vi "STOP.vi"(8 "error in (no error)":errorcluster, 11 "Stop in":refnum<class "Emulate.lvclass">) -> (0 "error out":errorcluster, 3 "Stop out":refnum<class "Emulate.lvclass">)   [LabVIEW 2019, in "Emulate.lvclass"]
uses:
  Emulate.lvclass
  C:/Users/elysium/Documents/dev/TRANCON/Classes/GeneralFunctionality/GeneralFunctionality.lvclass
  GeneralFunctionality/GeneralFunctionality.lvclass/GeneralFunctionality.ctl
  GeneralFunctionality/GeneralFunctionality.lvclass
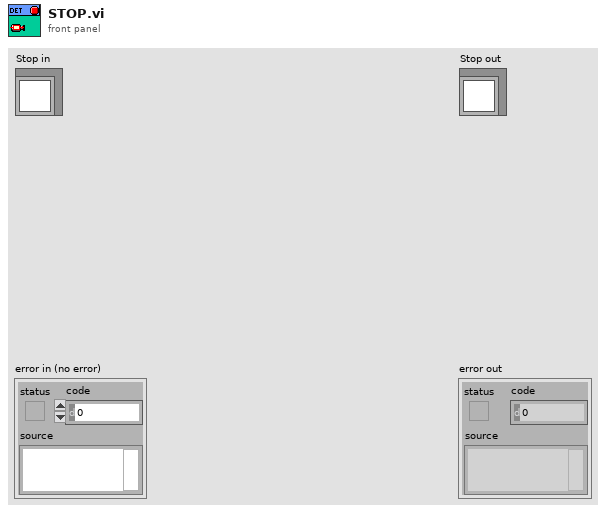
[diagram p1: front panel]
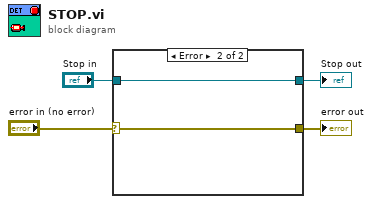
[diagram p0: block diagram]
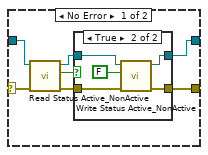
[diagram p2: hidden frame]
diagram:
  n1 = case shown="Error" "error in (no error)" {
    selector: "error in (no error)" -> [w6 w19]
    tunnel: "Stop in" -> [w9 w20]
    tunnel: [w8 w20] -> w3
    tunnel: [w7 w19] -> w2
    frame No Error {
      n2 = call "Read Status Active_NonActive.vi"("error in (no error)"=w6, "GeneralFunctionality in"=w9) -> ("error out"=w5:errorcluster, "Status Active/NonActive"=w10:bool, "GeneralFunctionality out"=w11:refnum<class "Emulate.lvclass">)  [unwired: 7 in]
      n3 = case shown="True" w10 {
        tunnel: [w13 w18] -> w8
        tunnel: w11 -> [w13 w16]
        tunnel: [w12 w15] -> w7
        tunnel: w5 -> [w12 w14]
        frame False {
        }
        frame True {
          n4 = call "Write Status Active_NonActive.vi"("error in (no error)"=w14, "Status Active/NonActive"=FALSE, "GeneralFunctionality in"=w16) -> ("error out"=w15:errorcluster, "GeneralFunctionality out"=w18:refnum<class "Emulate.lvclass">)  [unwired: 7 in]
        }
      }
    }
    frame Error {
    }
  }
  "error out" <- w2
  "Stop out" <- w3
